vi "Extrema of f(x1,x2).vi"(0 "End":dbl[](array[numeric])=[1.0, 1.0] format="%.2f", 1 "Start":dbl[](array[numeric])=[0.0, 0.0] format="%.2f", 2 "formula":string, 3 "Variables":string[](array[string])=["x1", "x2"], 4 "number of trials":i32) -> (6 "Minima":dbl[][](array[numeric]) format="%.2f", 7 "Maxima":dbl[][](array[numeric]) format="%.2f", 8 "error":i32, 9 "ticks":u32)   [LabVIEW 2010, in "NI_Gmath.lvlib"]
doc: "The algorithm looks for local extrema of a given function of two variables on a given rectangle. The absolute distance between two extrema must be equal to or greater than 1E-6 for the two vectors to register as different from each other."
uses:
  NI_Gmath.lvlib
panel:
  # "Example:\n\n Start: 0.0 and 0.0\n End: 1.0 and 1.0\n formula: 7*sin(x1)^2+cos(3*x2)^2  \n Variables: x1 and x2 \n number of trials: 5"
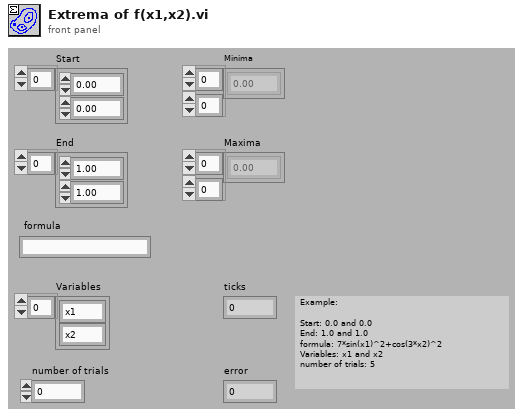
[diagram p1: front panel]
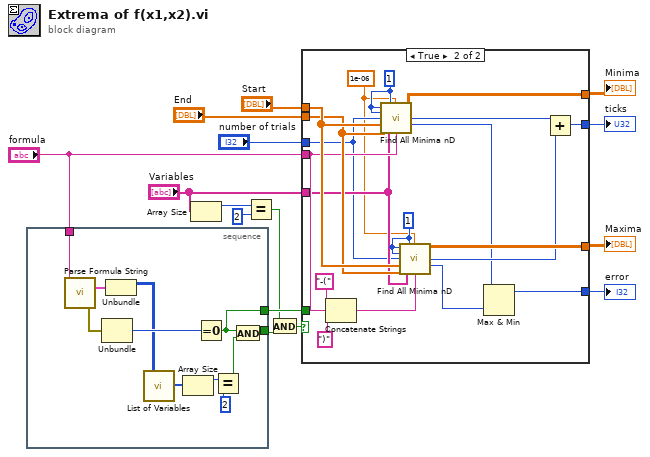
[diagram p0: block diagram]
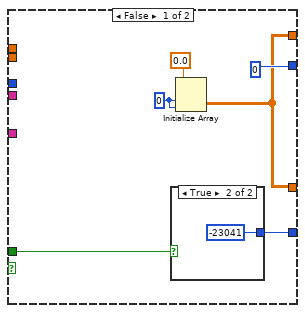
[diagram p2: hidden frame]
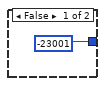
[diagram p3: hidden frame]
diagram:
  n1 = stacked-sequence {
    tunnel: [w26] -> w3
    tunnel: "formula" -> [w21]
    tunnel: [w18] -> w10
    frame #0 {
      n2 = call "Parse Formula String.vi"("formula"=w21) -> ("error out"=w20:errorcluster, "Parsed Formula"=w17:cluster{"Table":i32[][], "Y Values":dbl[]})  [unwired: 1 in]
      n3 = Unbundle(w20) -> ("code"=w19:i32)  [unwired: 2 out]
      n4 = Unbundle(w17) -> ("Table"=w16:i32[][])  [unwired: 1 out]
      n5 = call "List of Variables.vi"("Table"=w16) -> ("List of variables"=w22:i32[])
      n6 = Array Size(array=w22) -> (size(s)=w23:i32)
      n7 = Equal To 0?(x=w19) -> (x = 0?=w18:bool)
      n8 = Equal?(x=w23, y=2) -> (x = y?=w25:bool)
      n9 = And(x=w18, y=w25) -> (x .and. y?=w26:bool)
    }
  }
  n10 = Array Size(array="Variables") -> (size(s)=w5:i32)
  n11 = Equal?(x=w5, y=2) -> (x = y?=w1:bool)
  n12 = And(x=w1, y=w3) -> (x .and. y?=w2:bool)
  n13 = case shown="True" w2 {
    tunnel: [u32 0 w52] -> w15
    tunnel: [w29 w51] -> w14
    tunnel: [w29 w50] -> w13
    tunnel: "Start" -> [_ w47]
    tunnel: "End" -> [_ w46]
    tunnel: "Variables" -> [_ w43]
    tunnel: "formula" -> [_ w45]
    tunnel: "number of trials" -> [_ w40]
    tunnel: w10 -> [w28 _]
    tunnel: [w27 w38] -> w9
    frame False {
      w30 = 0
      n14 = case shown="True" w28 {
        tunnel: [-23001 -23041] -> w27
        frame False {
        }
        frame True {
        }
      }
      n15 = Initialize Array(0.0, w30, w30) -> (w29:dbl[][])
    }
    frame True {
      w35 = 1e-06
      w39 = u16 1
      w41 = u16 1
      n16 = Concatenate Strings("-(", w45, ")") -> (w44:string)
      n17 = call "Find All Minima nD.vi"("gradient method"=w41, "algorithm"=w41, "accuracy"=w35, "line minimum"=w41, "number of trials"=w40, "Start"=w47, "End"=w46, "X"=w43, "F(X)"=w45) -> ("X Values"=w51:dbl[][], "ticks"=w36:u32, "error"=w42:i32)  [unwired: 3 in, 1 out]
      n18 = call "Find All Minima nD.vi"("gradient method"=w39, "algorithm"=w39, "accuracy"=w35, "line minimum"=w39, "number of trials"=w40, "Start"=w47, "End"=w46, "X"=w43, "F(X)"=w44) -> ("X Values"=w50:dbl[][], "ticks"=w48:u32, "error"=w37:i32)  [unwired: 3 in, 1 out]
      n19 = Max & Min(x=w42, y=w37) -> (max(x,y)=w38:i32)  [unwired: 1 out]
      n20 = Add(x=w36, y=w48) -> (x+y=w52:u32)
    }
  }
  "ticks" <- w15
  "Minima" <- w14
  "Maxima" <- w13
  "error" <- w9
